vi "test.vi"(6 "Line Scan":bool, 7 "RIO Device":T2="RIO0", 8 "DMA Buffer Size\n(In Images)":u32=64 caption="DMA Buffer Size", 9 "Signal Mapping":T1(ring)=enum."Basler 10-tap", 10 "Image Height":u32=1024 max=65535, 11 "Image Width":u32=1280 max=65535 step=40) -> ()   [LabVIEW 2014]
uses:
  <vilib>/userdefined/High Color/nirio_resource_hc.ctl
  <vilib>/FPGAPlugInAG/PCIe-1473R/niLvFpga_Open_PCIe-1473R.vi
  <vilib>/rvi/interface/common/dynamic/niFpgaDynamicAddResources.vi
  <vilib>/FPGAPlugInAG/Dynamic/niLvFpga_Reset_Dynamic.vi
  <vilib>/Utility/error.llb/Error Cluster From Error Code.vi
  <vilib>/rvi/errors/niLvFpgaAdjustHostInterfaceError.vi
  <vilib>/FPGAPlugInAG/Dynamic/niLvFpga_Run_Dynamic.vi
  <vilib>/rvi/interface/common/niFpgaWaitOnOcc.vi
  <vilib>/FPGAPlugInAG/Dynamic/niLvFpga_Close_Dynamic.vi
  <vilib>/rvi/interface/nirviOpenFPGA/nirviOpenFPGA.xnode
  FPGA Bitfiles/10-Tap8-bitCamer_FPGATarget_10-Tap8-bitCamer_C490DC32.lvbitx
  <vilib>/rvi/interface/nirviMethod/nirviMethod.xnode
  <vilib>/rvi/interface/nirviReadWriteControl/nirviReadWriteControl.xnode
  <vilib>/rvi/interface/nirviCloseFPGA/nirviCloseFPGA.xnode
  NiFpgaLv.dll
  <vilib>/rvi/interface/Simulation/niFpgaSimulationCallBeginRW.vi
  <vilib>/FPGAPlugInAG/Dynamic/niLvFpga_ReadFifo_Dynamic.vi
  <vilib>/rvi/errors/niLvFpgaMergeErrorWithErrorCode.vi
  <vilib>/FPGAPlugInAG/Dynamic/niLvFpga_ConfigureFifo_Dynamic.vi
  <vilib>/FPGAPlugInAG/Dynamic/niLvFpga_StartFifo_Dynamic.vi
panel:
  in  "Start Serial Server":bool=TRUE
  out "DMA Write Timeout":bool
  in  "Stopped":bool
  out "Acq In Progress":bool
  in  "Acquire":bool
  in  "Stop":bool
  in  "Cancel":bool
  out "Initialized":bool
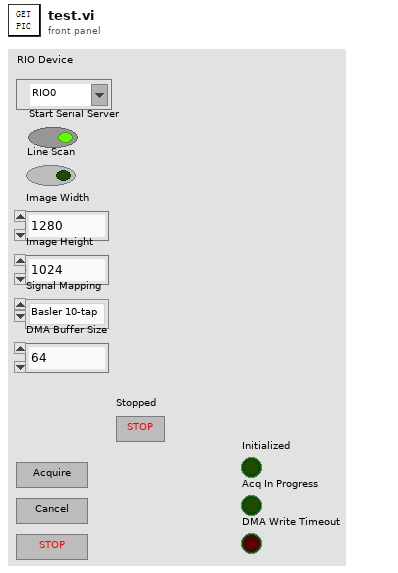
[diagram p1: front panel]
types:
  T1 = enum8{"Standard", "Basler 10-tap", "Vosskühler 10-tap"}
  T2 = typedef "nirio_resource_hc.ctl" = tag
  T3 = enum16{"big-endian, network order", "native, host order", "little-endian"}
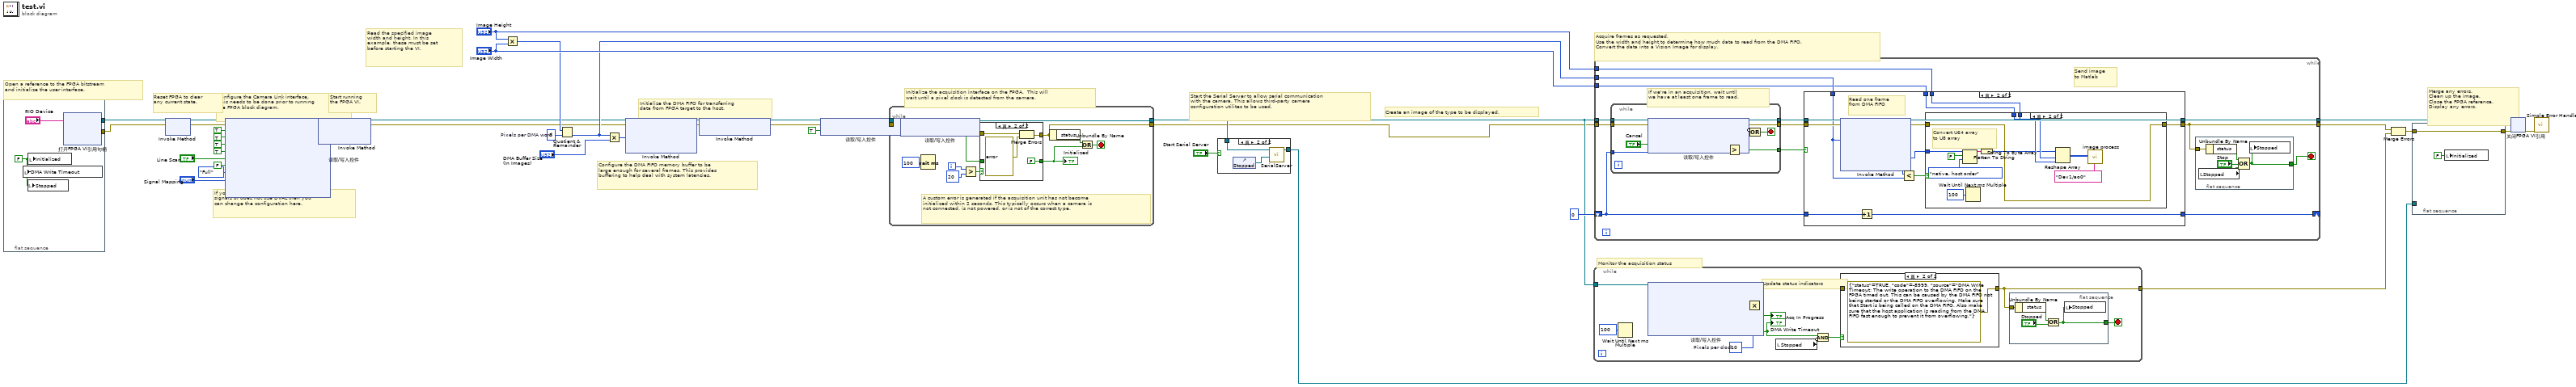
[diagram p0: block diagram]
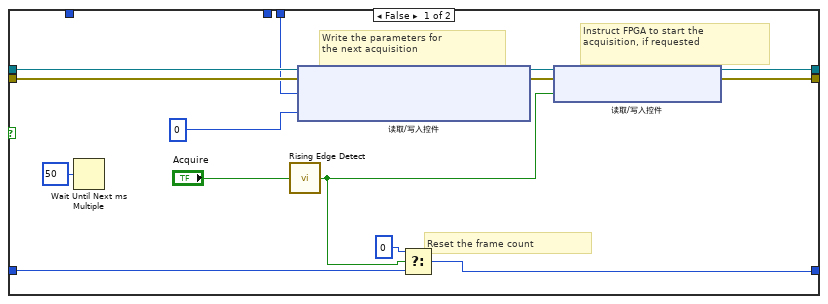
[diagram p4: hidden frame]
diagram:
  w6 = u32 8  # Pixels per DMA word
  # "If your camera outputs active-low enable\nsignals or does not use DVAL then you \ncan change the configuration here."
  # "Configure the DMA FIFO memory buffer to be\nlarge enough for several frames. This provides\nbuffering to help deal with system latencies."
  # "Start running\nthe FPGA VI."
  # "Reset FPGA to clear\nany current state."
  # "Read the specified image\nwidth and height. In this\nexample, these must be set\nbefore starting the VI."
  # "Merge any errors.\nClean up the image.\nClose the FPGA reference.\nDisplay any errors."
  # "Acquire frames as requested.\nUse the width and height to determine how much data to read from the DMA FIFO.\nConvert the data into a Vision Image for display."
  # "Monitor the acquisition status"
  # "Start the Serial Server to allow serial communication\nwith the camera. This allows third-party camera\nconfiguration utilites to be used."
  # "Create an image of the type to be displayed."
  # "Initialize the acquisition interface on the FPGA.  This will\nwait until a pixel clock is detected from the camera."
  # "Initialize the DMA FIFO for transferring\ndata from FPGA target to the host."
  # "Configure the Camera Link interface.\nThis needs to be done prior to running\nthe FPGA block diagram."
  # "Open a reference to the FPGA bitstream\nand initialize the user interface."
  n1 = flat-sequence {
    tunnel: [w43] -> w31
    tunnel: [w42] -> w41
    frame #0 {
      w45 = FALSE ("stop")
      n2 = local write "DMA Write Timeout"(w45) -> ()
      n3 = local write "Stopped"(w45) -> ()
      n4 = local write "Initialized"(w45) -> ()
      n5 = xnode "打开FPGA VI引用句柄"("资源名称"="RIO Device") -> ("FPGA VI引用输出"=w43:refnum<k20>, "错误输出"=w42:errorcluster)  [unwired: 1 in]
    }
  }
  n6 = xnode "Invoke Method"("FPGA VI引用输入"=w31, "错误输入"=w41) -> ("FPGA VI引用输出"=w20:refnum<k20>, "错误输出"=w23:errorcluster)
  n7 = xnode "读取/写入控件"("FPGA VI引用输入"=w20, "错误输入"=w23, "CL Config.FVAL Active High"=TRUE ("IO Module Config.CL FVAL Active High"), "CL Config.LVAL Active High"=TRUE ("IO Module Config.CL LVAL Active High"), "CL Config.DVAL Active High"=TRUE ("IO Module Config.CL DVAL Active High"), "CL Config.Spare Active High"=TRUE ("IO Module Config.CL Spare Active High"), "CL Config.Line Scan"="Line Scan", "Acq Control.Ignore DVAL"=FALSE ("CL Config.Line Scan"), "CL Config.Configuration"=enum8{"Base", "Medium", "Full"}."Full", "CL Config.Signal Mapping"="Signal Mapping") -> ("FPGA VI引用输出"=w24:refnum<k20>, "错误输出"=w22:errorcluster)
  n8 = xnode "Invoke Method"("FPGA VI引用输入"=w24, "错误输入"=w22) -> ("FPGA VI引用输出"=w3:refnum<k20>, "错误输出"=w2:errorcluster)  [unwired: 1 in]
  n9 = Multiply(x="Image Height", y="Image Width") -> (x*y=w5:u32)
  n10 = Quotient & Remainder(x=w5, y=w6) -> (floor(x/y)=w4:u32)  [unwired: 1 out]
  n11 = Multiply(x=w4, y="DMA Buffer Size\n(In Images)") -> (x*y=w14:u32)
  n12 = xnode "Invoke Method"("FPGA VI引用输入"=w3, "错误输入"=w2, "请求的深度"=w14) -> ("FPGA VI引用输出"=w30:refnum<k20>, "错误输出"=w29:errorcluster)  [unwired: 1 out]
  n13 = xnode "Invoke Method"("FPGA VI引用输入"=w30, "错误输入"=w29) -> ("FPGA VI引用输出"=w15:refnum<k20>, "错误输出"=w28:errorcluster)
  n14 = xnode "读取/写入控件"("FPGA VI引用输入"=w15, "错误输入"=w28, "Acq Control.Initialize"=TRUE ("Arm Acquisition")) -> ("FPGA VI引用输出"=w40:refnum<k20>, "错误输出"=w39:errorcluster)
  n15 = while {
    tunnel: w40 -> [w53]
    tunnel: w39 -> [w52]
    tunnel: [w51] -> w11
    tunnel: [w55] -> w1
    i -> [w47]
    stop <- w58 stop-if-true
    # "A custom error is generated if the acquisition unit has not become\ninitialized within 2 seconds. This typically occurs when a camera is\nnot connected, is not powered, or is not of the correct type."
    n16 = xnode "读取/写入控件"("FPGA VI引用输入"=w53, "错误输入"=w52) -> ("FPGA VI引用输出"=w51:refnum<k20>, "错误输出"=w50:errorcluster, "Acq Status.Initialized"=w49:bool)
    n17 = Wait (ms)(milliseconds to wait=u32 100) -> ()  [unwired: 1 out]
    n18 = Greater?(x=w47, y=20) -> (0:w48:bool)
    n19 = case shown="真" w48 {
      tunnel: [w60 FALSE] -> w54
      tunnel: w49 -> [w60 _]
      tunnel: w50 -> [w59 w62]
      tunnel: [w59 w64] -> w55
      frame False {
      }
      frame True {
        n20 = Merge Errors(w62, errorcluster {"status"=TRUE, "code"=-8999, "source"="Acquisition Initialization: This error typically occurs when a camera is not properly connected, is not powered, or is not of the correct type."} ("error in")) -> (w64:errorcluster)
      }
    }
    "Initialized" <- w54
    n21 = Unbundle By Name(w55) -> ("status"=w57:bool)
    n22 = Or(x=w57, y=w54) -> (x .or. y?=w58:bool)
  }
  n23 = case shown="真" "Start Serial Server" {
    tunnel: [_ w65] -> w32
    tunnel: w11 -> [_ w66]
    frame False {
    }
    frame True {
      n24 = control-ref of="Stopped"() -> (w67:refnum<vi>)
      n25 = call "SerialServer.vi"("Stop Refnum"=w67, "FPGA VI Reference In"=w66) -> ("FPGA VI Reference Out"=w65:refnum<k20>)  [unwired: 5 in]
    }
  }
  n26 = while {
    tunnel: w11 -> [w75]
    tunnel: [w78] -> w25
    stop <- w77 stop-if-true
    w71 = u32 10  # Pixels per clock
    # "Update status indicators"
    n27 = Wait Until Next ms Multiple(millisecond multiple=u32 100) -> ()  [unwired: 1 out]
    n28 = xnode "读取/写入控件"("FPGA VI引用输入"=w75) -> ("错误输出"=w74:errorcluster, "Acq Status.Clocks Per Line"=w72:u32, "Acq Status.Acq In Progress"=→"Acq In Progress":bool, "Acq Status.DMA Write Timeout"=w69:bool)  [unwired: 1 in, 3 out]
    "DMA Write Timeout" <- w69
    n29 = Multiply(x=w72, y=w71) -> ()  [unwired: 1 out]
    n30 = local read "Stopped"() -> (w68:bool)
    n31 = Compound Arithmetic op=AND(w69, invert w68) -> (w70:bool)
    n32 = case shown="真" w70 {
      tunnel: w74 -> [w83 _]
      tunnel: [w83 errorcluster {"status"=TRUE, "code"=-8999, "source"="DMA Write Timeout: The write operation to the DMA FIFO on the FPGA timed out. This can be caused by the DMA FIFO not being started or the DMA FIFO overflowing. Make sure that Start is being called on the DMA FIFO. Also make sure that the host application is reading from the DMA FIFO fast enough to prevent it from overflowing."} ("error out")] -> w78
      frame False {
      }
      frame True {
      }
    }
    n33 = flat-sequence {
      tunnel: w78 -> [w82]
      tunnel: [w80] -> w77
      frame #0 {
        n34 = Unbundle By Name(w82) -> ("status"=w81:bool)
        n35 = Or(x=w81, y="Stopped") -> (x .or. y?=w80:bool)
        n36 = local write "Stopped"(w80) -> ()
      }
    }
  }
  n37 = while {
    tunnel: w11 -> [w93]
    tunnel: w1 -> [w92]
    tunnel: w4 -> [w97]
    tunnel: "Image Height" -> [w96]
    tunnel: "Image Width" -> [w95]
    tunnel: [w86] -> w26
    tunnel: [w94] -> w38
    shift-right: [w88] -> _
    shift-left: u32 0 -> [w87]
    stop <- w85 stop-if-true
    # "Send image\nto Matlab"
    # "If we're in an acquisition, wait until\nwe have at least one frame to read."
    n38 = while {
      tunnel: w93 -> [w109]
      tunnel: w92 -> [w108]
      tunnel: [w106] -> w91
      tunnel: [w107] -> w90
      tunnel: w87 -> [w112]
      tunnel: [w110] -> w89
      stop <- w111 stop-if-true
      n39 = xnode "读取/写入控件"("FPGA VI引用输入"=w109, "错误输入"=w108, "Acq Control.Cancel Acq"="Cancel") -> ("FPGA VI引用输出"=w107:refnum<k20>, "错误输出"=w106:errorcluster, "Acq Status.Acq In Progress"=w105:bool, "Acq Status.Frames Acq'd"=w104:u32)
      n40 = Greater?(x=w104, y=w112) -> (0:w110:bool)
      n41 = Compound Arithmetic op=OR(invert w105, w110) -> (w111:bool)
    }
    n42 = case shown="真" w89 {
      tunnel: w90 -> [w123 w134]
      tunnel: w91 -> [w122 w133]
      tunnel: w97 -> [_ w127]
      tunnel: w96 -> [w116 w139]
      tunnel: w95 -> [_ w138]
      tunnel: [w118 w136] -> w86
      tunnel: [w121 w135] -> w94
      tunnel: w87 -> [w124 w132]
      tunnel: [w126 w131] -> w88
      frame False {
        # "Reset the frame count"
        # "Instruct FPGA to start the\nacquisition, if requested"
        # "Write the parameters for\nthe next acquisition"
        n43 = Wait Until Next ms Multiple(millisecond multiple=u32 50) -> ()  [unwired: 1 out]
        n44 = call "Rising Edge Detect.vi"("Input"="Acquire") -> ("Pulse"=w114:bool)  [unwired: 4 in]
        n45 = xnode "读取/写入控件"("FPGA VI引用输入"=w123, "错误输入"=w122, "Acq Control.Line Scan Height"=w116, "Acq Control.Frames To Acq"=0) -> ("FPGA VI引用输出"=w120:refnum<k20>, "错误输出"=w119:errorcluster)
        n46 = Select(t=u32 0, s=w114, f=w124) -> (s? t:f=w126:u32)
        n47 = xnode "读取/写入控件"("FPGA VI引用输入"=w120, "错误输入"=w119, "Acq Control.Acquire"=w114) -> ("FPGA VI引用输出"=w121:refnum<k20>, "错误输出"=w118:errorcluster)
      }
      frame True {
        # "Read one frame\nfrom DMA FIFO"
        n48 = xnode "Invoke Method"("FPGA VI引用输入"=w134, "错误输入"=w133, "元素数量"=w127) -> ("FPGA VI引用输出"=w135:refnum<k20>, "错误输出"=w137:errorcluster, "数据"=w130:u64[], "剩余元素"=w128:u32)  [unwired: 1 in]
        n49 = Increment(x=w132) -> (x+1=w131:u32)
        n50 = Less?(x=w128, y=w127) -> (x < y?=w129:bool)
        n51 = case shown="真" w129 {
          tunnel: w139 -> [_ w151]
          tunnel: w138 -> [_ w150]
          tunnel: w137 -> [w140 w144]
          tunnel: [w140 w144] -> w136
          tunnel: w130 -> [_ w148]
          frame False {
            # "Do not display the image if we're falling behind in the acquisition."
          }
          frame True {
            # "Convert U64 array\nto U8 array"
            n52 = Flatten To String(anything=w148, prepend array or string size? (T)=FALSE, byte order (0:big-endian, network order)=T3."native, host order") -> (data string=w146:string)  [unwired: 1 in, 2 out]
            n53 = Wait Until Next ms Multiple(millisecond multiple=u32 100) -> ()  [unwired: 1 out]
            n54 = String To Byte Array(string=w146) -> (unsigned byte array=w145:u8[])
            n55 = Reshape Array(w145, w151, w150) -> (w143:u8[][])
            n56 = call "image process.vi"("物理通道"=tag "Dev1/ao0", "输出数组"=w143) -> ()  [unwired: 10 in]
          }
        }
      }
    }
    n57 = flat-sequence {
      tunnel: w86 -> [w100]
      tunnel: [w99] -> w85
      frame #0 {
        n58 = local read "Stopped"() -> (w98:bool)
        n59 = Unbundle By Name(w100) -> ("status"=w101:bool)
        n60 = Compound Arithmetic op=OR(w101, "Stop", w98) -> (w99:bool)
        n61 = local write "Stopped"(w99) -> ()
      }
    }
  }
  n62 = Merge Errors(w26, w25) -> (w27:errorcluster)
  n63 = flat-sequence {
    tunnel: w27 -> [w153]
    tunnel: [w153] -> w35
    tunnel: w32 -> [_]
    frame #0 {
      n64 = local write "Initialized"(FALSE ("Module Enabled")) -> ()
    }
  }
  n65 = xnode "关闭FPGA VI引用"("FPGA VI引用输入"=w38, "错误输入"=w35) -> ("错误输出"=w33:errorcluster)
  n66 = call <vilib>:"Simple Error Handler.vi"("error in (no error)"=w33) -> ()  [unwired: 4 in, 5 out]
